vi "global-Broadcast Cache Change Flag.vi"() -> ()   [LabVIEW 2014, in "JKI State Machine++.lvlib"]
uses:
  JKI State Machine++.lvlib
panel:
  in  "global-Broadcast Cache Change Flag":u32
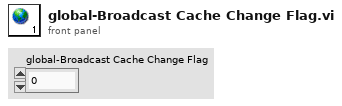
[diagram p1: front panel]
diagram:
